vi "Configure.vi"(8 "error in (no error)":errorcluster, 9 "Digital Configuration Parameters":T1, 10 "External Control?":bool) -> (0 "error out":errorcluster, 3 "Binary Valve out":refnum<class "Binary Valve.lvclass">)   [LabVIEW 2021, in "Binary Valve.lvlib" / "Binary Valve.lvclass"]
uses:
  Binary Valve.lvclass
  <vilib>/NathanCo/Digital-Tasks/Utilities/Digital Configuration Parameters.ctl
  Binary Valve.lvclass/Binary Valve.ctl
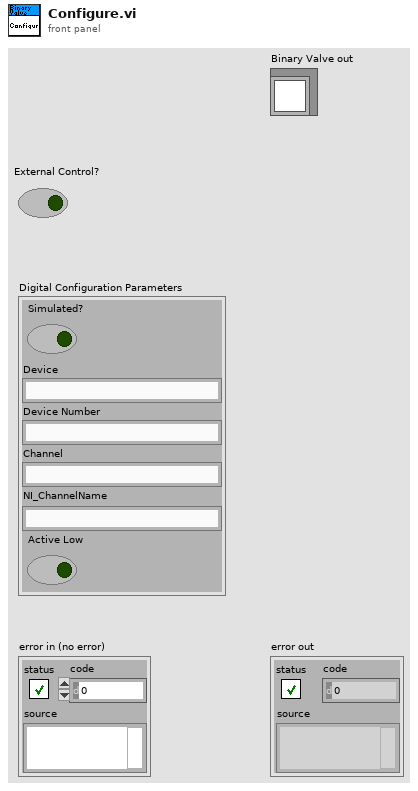
[diagram p1: front panel]
types:
  T1 = typedef "Digital Configuration Parameters.ctl" = cluster{"Simulated?":bool, "Device":string, "Device Number":string, "Channel":string, "NI_ChannelName":string, "Active Low":bool}
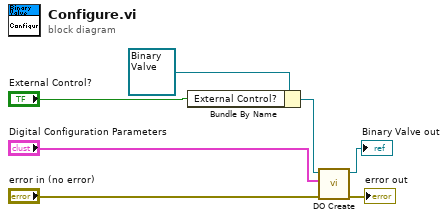
[diagram p0: block diagram]
diagram:
  n1 = Bundle By Name(cluster=refnum<class "Binary Valve.lvclass"> refnum ("Valve.lvlib:Valve.lvclass"), "External Control?"="External Control?") -> (w6:refnum<class "Binary Valve.lvclass">)
  n2 = call "DO Create.vi"("error in (no error)"="error in (no error)", "Digital Configuration Parameters"="Digital Configuration Parameters", "Binary Valve in"=w6) -> ("error out"=→"error out":errorcluster, "Binary Valve out"=→"Binary Valve out":refnum<class "Binary Valve.lvclass">)  [unwired: 7 in]
